vi "RT Driver VI.vi"(7 "Operation":T1, 11 "Device Reference in":T2 format="%.0x") -> (0 "Error Code":i32)   [LabVIEW 2016, in "UDP-Custom-Device Engine.lvlib"]
uses:
  UDP-Custom-Device Engine.lvlib
  <vilib>/NI Veristand/Custom Device API/Custom Device Item Ref.ctl
  <vilib>/NI Veristand/Custom Device API/Hardware Interface Driver VI Operation.ctl
  Types/Engine - RTStateVariables.ctl
  <vilib>/NI/NIVS Inline Async API/_VS Inline Async API/VS Inline Async API/VS Inline Async API.lvclass
  Shared/Compiled.Settings.ctl
  Shared/Types/Shared - Rx.PacketInfo.ctl
  Shared/Types/Shared - Channel Data Type.ctl
  Shared/Types/Shared - Buffered.PacketInfo.ctl
  Shared/Types/Shared - Tx.PacketInfo.ctl
  Shared/Types/Shared - Header Details.ctl
  Shared/Types/Shared - Duplex Settings.ctl
  <vilib>/NI/NIVS Inline Async API/_Data Access Engine/Data Access Engine/Types/Write.DVR.ctl
  <vilib>/NI/NIVS Inline Async API/_Data Access Engine/Access Type Classes/Write/Write.lvclass
  <vilib>/NI/NIVS Inline Async API/_Data Access Engine/Data Access Engine/Types/Read.DVR.ctl
  <vilib>/NI/NIVS Inline Async API/_Data Access Engine/Access Type Classes/Read/Read.lvclass
  <vilib>/NI/NIVS Inline Async API/_VS Inline Async API/VS Inline Async API/VS Inline Async API.lvclass/VS Inline Async API.ctl
  <vilib>/NI/NIVS Inline Async API/_Data Access Engine/Data Access Engine/Data Access Engine.lvclass/Data Access Engine.ctl
  <vilib>/NI/NIVS Inline Async API/_Data Access Engine/Access Type Classes/Write/Write.lvclass/Write.ctl
  <vilib>/NI/NIVS Inline Async API/_Data Access Engine/Access Type Classes/ReadWrite/ReadWrite.lvclass/ReadWrite.ctl
  <vilib>/NI/NIVS Inline Async API/_Data Access Engine/Access Type Classes/Read/Read.lvclass/Read.ctl
  <vilib>/NI/NIVS Inline Async API/_Data Access Engine/Data Access Engine/Methods/Data.Engine.Read Data from HW.vi
  <vilib>/NI/NIVS Inline Async API/_VS Inline Async API/Error Handling Process/SubVIs/Error.GetError.vi
  <vilib>/NI/NIVS Inline Async API/_Data Access Engine/Data Access Engine/Methods/Data.Engine.Write Data to HW.vi
  <vilib>/NI/NIVS Inline Async API/_Data Access Engine/Access Type Classes/ReadWrite/ReadWrite.EngineData.vi
  <vilib>/NI/NIVS Inline Async API/_Data Access Engine/Access Type Classes/Write/Write.EngineData.vi
  <vilib>/NI/NIVS Inline Async API/_Data Access Engine/Access Type Classes/Read/Read.EngineData.vi
  <vilib>/NI Veristand/Custom Device API/NI VeriStand - Get Channel Value by Data Reference.vi
  <vilib>/NI Veristand/Custom Device API/NI VeriStand - Set Channel Value by Data Reference.vi
  <vilib>/NI Veristand/Custom Device API/NI VeriStand - Get Channel Values by Block Data Reference.vi
  Run/UDP Buffered Rx Process.vi
  Run/UDP Buffered Tx Process.vi
  <vilib>/NI Veristand/Custom Device API/Global Data Refs.vi
  <vilib>/NI VeriStand/Custom Device Tools/Custom Device Utility Library/Custom Device Utility Library.lvlib
  Shared/UDP-Custom-Device Shared.lvlib
  <vilib>/NI/NIVS Inline Async API/_Data Access Engine/Data Access Engine/Data Access Engine.lvclass
  <vilib>/NI VeriStand/Custom Device API/Custom Device API.lvlib
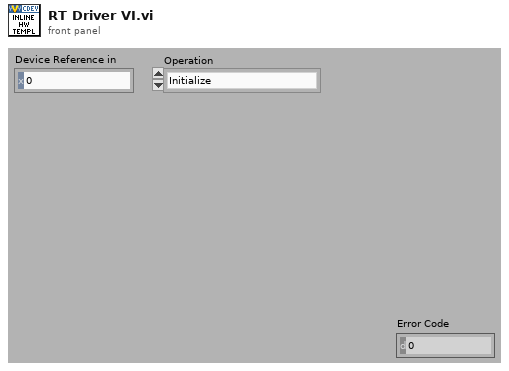
[diagram p1: front panel]
types:
  T1 = typedef "Custom Device API.lvlib/Hardware Interface Driver VI Operation.ctl" = enum16{"Initialize", "Start", "Read Data from HW", "Write Data to HW", "Close"}
  T2 = typedef "Custom Device API.lvlib/Custom Device Item Ref.ctl" = u64
  T3 = typedef "UDP-Custom-Device Engine.lvlib/Engine - RTStateVariables.ctl" = cluster{"Async":refnum<class "VS Inline Async API.lvclass">, "Settings":T4, "Connection ID":refnum<k16>, "Rx FIFO Ref":T11, "Tx FIFO Ref":T12}
  T4 = typedef "UDP-Custom-Device Shared.lvlib/Compiled.Settings.ctl" = cluster{"Name":string, "Tx Enabled?":bool, "Rx Enabled?":bool, "Rx Packet Info":T5[], "Tx Packet Info":T8[], "Duplex Packets":T10[]}
  T5 = typedef "UDP-Custom-Device Shared.lvlib/Shared - Rx.PacketInfo.ctl" = cluster{"Packet Name":string, "Packet ID":i32, "Timeout":i32, "Rx IP Address":string, "Rx Port":u16, "Endianness":u16, "Multicast":bool, "Multicast IP Address":string, "Diagnostics En?":bool, "Header Info":bool[], "Channel Data Types":T6[], "Buffered Packet Info":T7}
  T6 = typedef "UDP-Custom-Device Shared.lvlib/Shared - Channel Data Type.ctl" = enum16{"Boolean", "Single", "Double", "I8", "I16", "I32", "I64", "U8", "U16", "U32", "U64"}
  T7 = typedef "UDP-Custom-Device Shared.lvlib/Shared - Buffered.PacketInfo.ctl" = cluster{"Buffer Size":i32, "External Buffer":bool, "Prepend Header":bool, "Is Buffered":bool}
  T8 = typedef "UDP-Custom-Device Shared.lvlib/Shared - Tx.PacketInfo.ctl" = cluster{"Packet Name":string, "Packet ID":i32, "Decimation":u16, "Destination IP Address":string, "Destination Port":u16, "Local IP Address":string, "Local Port":u16, "Endianness":u16, "Always Transmit":bool, "TTL":u16, "Multicast":bool, "Multicast IP Address":string, "Header Info":bool[], "PCL Period":u32, "Channel Data Types":T6[], "Header Details":T9, "Buffered Packet Info":T7}
  T9 = typedef "UDP-Custom-Device Shared.lvlib/Shared - Header Details.ctl" = cluster{"Packet Size":u16, "Protocol Revision":u8, "System Definition Version":u64, "Source Node Name":string, "Packet ID":u32, "Number of Channels":u32, "Static Header Size":u16, "Total Header Size":u16}
  T10 = typedef "UDP-Custom-Device Shared.lvlib/Shared - Duplex Settings.ctl" = cluster{"Transmit Packet ID":i32, "Receive Packet ID":i32, "Multicast":bool, "Multicast Address":string, "IP Address":string, "Port":u16, "TTL":u16, "Duplex Connection":refnum<k16>}
  T11 = typedef "Data Access Engine.lvlib/Data Access Engine.lvclass/Write.DVR.ctl" = refnum<data-value>
  T12 = typedef "Data Access Engine.lvlib/Data Access Engine.lvclass/Read.DVR.ctl" = refnum<data-value>
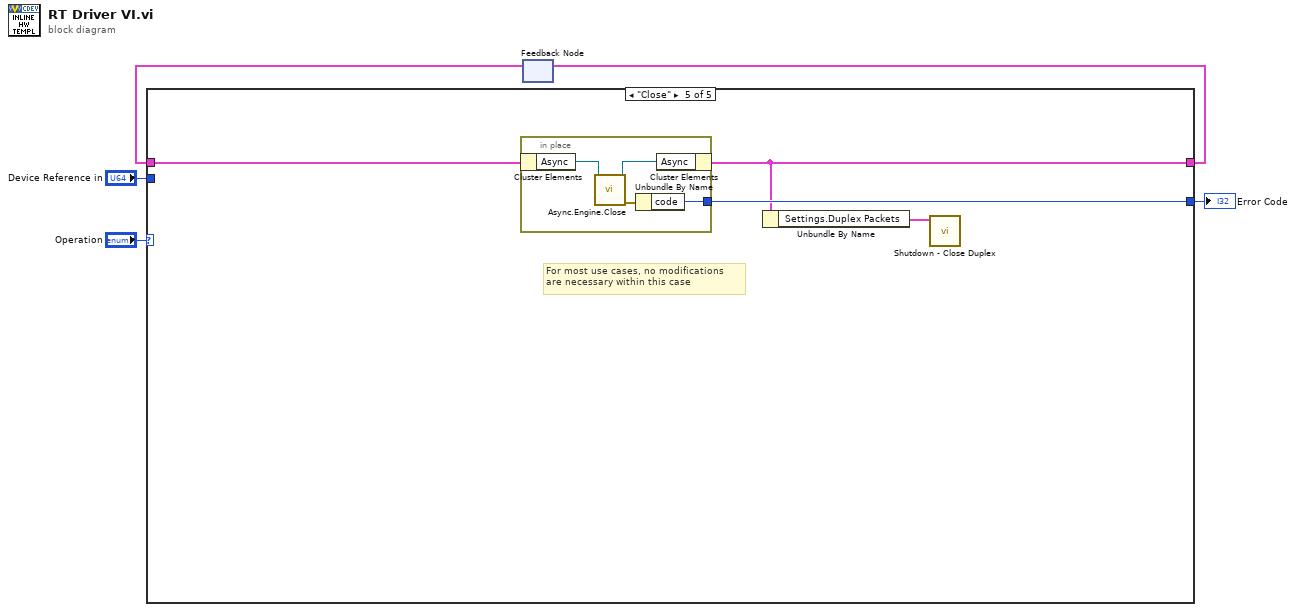
[diagram p0: block diagram]
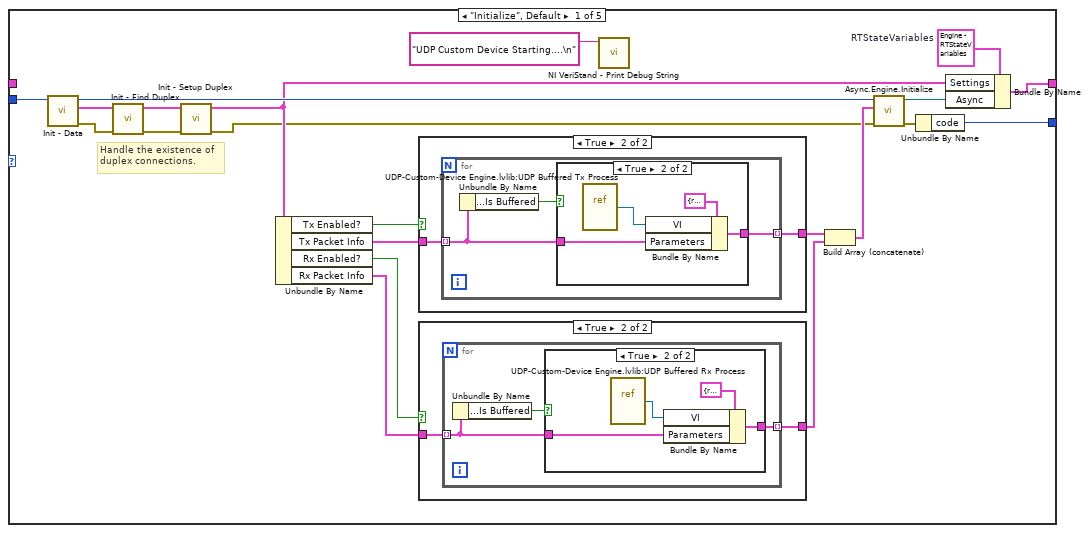
[diagram p2: hidden frame]
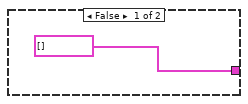
[diagram p3: hidden frame]
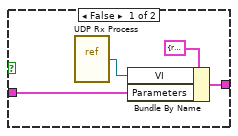
[diagram p4: hidden frame]
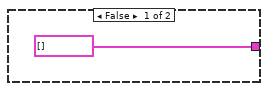
[diagram p5: hidden frame]
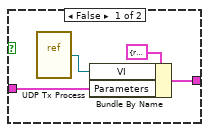
[diagram p6: hidden frame]
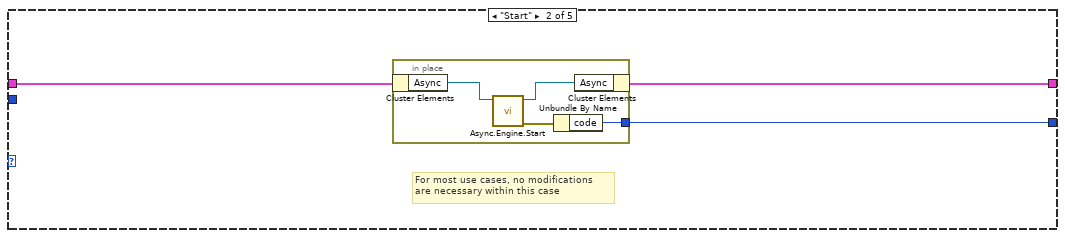
[diagram p7: hidden frame]
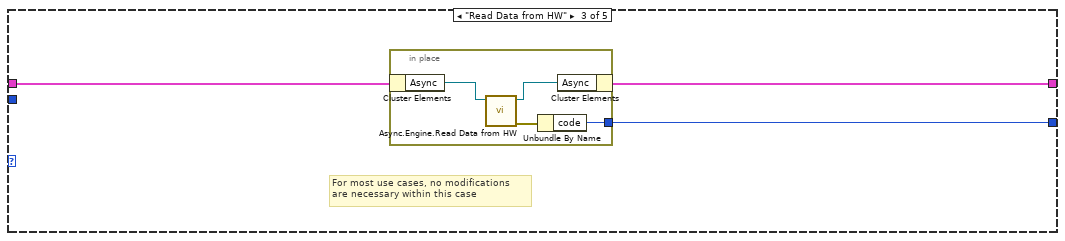
[diagram p8: hidden frame]
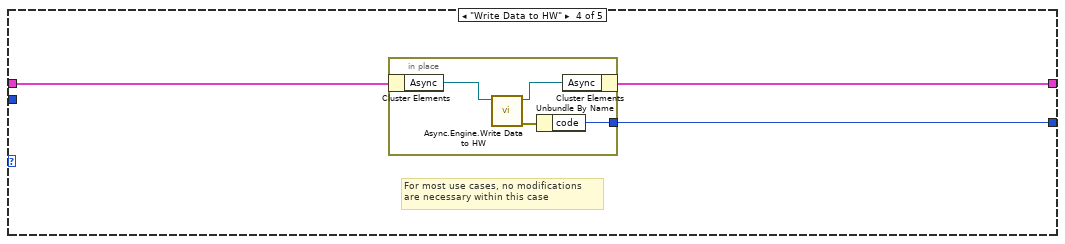
[diagram p9: hidden frame]
diagram:
  n1 = feedback #1() -> (w3:T3)  [unwired: 1 out]
  n2 = case shown="\"Close\"" "Operation" {
    tunnel: [w24 w56 w62 w69 w77] -> w4
    tunnel: w3 -> [_ w57 w64 w70 w79]
    tunnel: "Device Reference in" -> [w21 _ _ _ _]
    tunnel: [w26 w55 w63 w71 w78] -> w1
    frame "Initialize", Default {
      w23 = T3 {"Async"=refnum, "Settings"={"Name"="", "Tx Enabled?"=FALSE, "Rx Enabled?"=FALSE, "Rx Packet Info"=[], "Tx Packet Info"=[], "Duplex Packets"=[]}, "Connection ID"=refnum, "Rx FIFO Ref"=refnum, "Tx FIFO Ref"=refnum}  # RTStateVariables
      # "Handle the existence of\nduplex connections."
      n3 = call "Init - Data.vi"("Device Reference in"=w21) -> ("error out"=w10:errorcluster, "Compiled.Settings"=w11:T4, "Device Reference out"=w17:T2)  [unwired: 8 in]
      n4 = call "Init - Find Duplex.vi"("error in (no error)"=w10, "Compiled.Settings in"=w11) -> ("error out"=w7:errorcluster, "Compiled.Settings out"=w9:T4)  [unwired: 8 in]
      n5 = call "Init - Setup Duplex.vi"("error in (no error)"=w7, "Compiled.Settings in"=w9) -> ("error out"=w6:errorcluster, "Compiled.Settings out"=w8:T4)  [unwired: 8 in]
      n6 = Unbundle By Name(w8) -> ("Tx Enabled?"=w20:bool, "Tx Packet Info"=w19:T8[], "Rx Enabled?"=w12:bool, "Rx Packet Info"=w18:T5[])
      n7 = case shown="True" w20 {
        tunnel: w19 -> [_ w43]
        tunnel: [cluster{"VI":refnum<vi>, "Parameters":variant}[] [] w42] -> w14
        frame False {
        }
        frame True {
          n8 = for {
            tunnel: w43 -> [w45] mode=indexing
            tunnel: [w46] -> w42 mode=indexing
            n9 = Unbundle By Name(w45) -> ("Buffered Packet Info.Is Buffered"=w44:bool)
            n10 = case shown="True" w44 {
              tunnel: [w48 w53] -> w46
              tunnel: w45 -> [w47 w52]
              frame False {
                n11 = vi-ref "UDP Tx Process.vi"() -> (w49:refnum<vi>)
                n12 = Bundle By Name(cluster=cluster{"VI":refnum<vi>, "Parameters":variant} {"VI"=refnum, "Parameters"=variant} ("Process"), "VI"=w49, "Parameters"=w47) -> (w48:cluster{"VI":refnum<vi>, "Parameters":variant})
              }
              frame True {
                n13 = vi-ref "UDP-Custom-Device Engine.lvlib:UDP Buffered Tx Process.vi"() -> (w51:refnum<vi>)
                n14 = Bundle By Name(cluster=cluster{"VI":refnum<vi>, "Parameters":variant} {"VI"=refnum, "Parameters"=variant} ("Process"), "VI"=w51, "Parameters"=w52) -> (w53:cluster{"VI":refnum<vi>, "Parameters":variant})
              }
            }
          }
        }
      }
      n15 = case shown="True" w12 {
        tunnel: w18 -> [_ w29]
        tunnel: [cluster{"VI":refnum<vi>, "Parameters":variant}[] [] w28] -> w13
        frame False {
        }
        frame True {
          n16 = for {
            tunnel: w29 -> [w31] mode=indexing
            tunnel: [w32] -> w28 mode=indexing
            n17 = Unbundle By Name(w31) -> ("Buffered Packet Info.Is Buffered"=w30:bool)
            n18 = case shown="True" w30 {
              tunnel: [w35 w39] -> w32
              tunnel: w31 -> [w33 w37]
              frame False {
                n19 = vi-ref "UDP Rx Process.vi"() -> (w36:refnum<vi>)
                n20 = Bundle By Name(cluster=cluster{"VI":refnum<vi>, "Parameters":variant} {"VI"=refnum, "Parameters"=variant} ("Process"), "VI"=w36, "Parameters"=w33) -> (w35:cluster{"VI":refnum<vi>, "Parameters":variant})
              }
              frame True {
                n21 = vi-ref "UDP-Custom-Device Engine.lvlib:UDP Buffered Rx Process.vi"() -> (w40:refnum<vi>)
                n22 = Bundle By Name(cluster=cluster{"VI":refnum<vi>, "Parameters":variant} {"VI"=refnum, "Parameters"=variant} ("Process"), "VI"=w40, "Parameters"=w37) -> (w39:cluster{"VI":refnum<vi>, "Parameters":variant})
              }
            }
          }
        }
      }
      n23 = call <vilib>:"NI VeriStand - Print Debug String.vi"("Message"="UDP Custom Device Starting....\n") -> ()  [unwired: 10 in, 1 out]
      n24 = Build Array (concatenate)(w14, w13) -> (w16:cluster{"VI":refnum<vi>, "Parameters":variant}[])
      n25 = call <vilib>:"Async.Engine.Initialize.vi"("error in (no error)"=w6, "Processes"=w16, "Custom Device Ref"=w17) -> ("error out"=w15:errorcluster, "Async"=w25:refnum<class "VS Inline Async API.lvclass">)  [unwired: 7 in]
      n26 = Unbundle By Name(w15) -> ("code"=w26:i32)
      n27 = Bundle By Name(cluster=w23, "Settings"=w8, "Async"=w25) -> (w24:T3)
    }
    frame "Start" {
      # "For most use cases, no modifications \nare necessary within this case"
      n28 = in-place {
        in-place-border: [w58] -> w55
        n29 = in-place-cluster #2(w57) -> ("Async"=w61:refnum<class "VS Inline Async API.lvclass">)
        n30 = call <vilib>:"Async.Engine.Start.vi"("VS Inline Async API in"=w61) -> ("error out"=w59:errorcluster, "VS Inline Async API out"=w60:refnum<class "VS Inline Async API.lvclass">)  [unwired: 9 in]
        n31 = Unbundle By Name(w59) -> ("code"=w58:i32)
        n32 = in-place-cluster #2("Async"=w60) -> (w56:T3)
      }
    }
    frame "Read Data from HW" {
      # "For most use cases, no modifications \nare necessary within this case"
      n33 = in-place {
        in-place-border: [w66] -> w63
        n34 = in-place-cluster #3(w64) -> ("Async"=w68:refnum<class "VS Inline Async API.lvclass">)
        n35 = call <vilib>:"Async.Engine.Read Data from HW.vi"("Async in"=w68) -> ("error out"=w65:errorcluster, "Async out"=w67:refnum<class "VS Inline Async API.lvclass">)  [unwired: 9 in]
        n36 = Unbundle By Name(w65) -> ("code"=w66:i32)
        n37 = in-place-cluster #3("Async"=w67) -> (w62:T3)
      }
    }
    frame "Write Data to HW" {
      # "For most use cases, no modifications \nare necessary within this case"
      n38 = in-place {
        in-place-border: [w75] -> w71
        n39 = in-place-cluster #4(w70) -> ("Async"=w73:refnum<class "VS Inline Async API.lvclass">)
        n40 = call <vilib>:"Async.Engine.Write Data to HW.vi"("VS Inline Async API in"=w73) -> ("error out"=w74:errorcluster, "VS Inline Async API out"=w72:refnum<class "VS Inline Async API.lvclass">)  [unwired: 9 in]
        n41 = Unbundle By Name(w74) -> ("code"=w75:i32)
        n42 = in-place-cluster #4("Async"=w72) -> (w69:T3)
      }
    }
    frame "Close" {
      # "For most use cases, no modifications \nare necessary within this case"
      n43 = in-place {
        in-place-border: [w81] -> w78
        n44 = in-place-cluster #5(w79) -> ("Async"=w83:refnum<class "VS Inline Async API.lvclass">)
        n45 = call <vilib>:"Async.Engine.Close.vi"("Async in"=w83) -> ("error out"=w80:errorcluster, "Async out"=w82:refnum<class "VS Inline Async API.lvclass">)  [unwired: 9 in]
        n46 = Unbundle By Name(w80) -> ("code"=w81:i32)
        n47 = in-place-cluster #5("Async"=w82) -> (w77:T3)
      }
      n48 = Unbundle By Name(w77) -> ("Settings.Duplex Packets"=w76:T10[])
      n49 = call "Shutdown - Close Duplex.vi"("Duplex Packets"=w76) -> ()  [unwired: 10 in, 1 out]
    }
  }
  "Error Code" <- w1
  n50 = feedback-in #1(w4) -> ()
